vi "Dialog_LogPack (SubVI).vi"() -> ()   [LabVIEW 2017]
uses:
  <vilib>/Utility/miscctls.llb/LVRowAndColumnTypeDef.ctl
  GlobalLog.vi
  <vilib>/Utility/file.llb/Write Delimited Spreadsheet (string).vi
panel:
  in  "Export":bool
  out "Slide":u8(slide) scale=0.0..100.0
  in  "Reload":bool
  in  "Cancel":bool
  in  "OK":bool
  out "Table":string[][](table) caption="Принятые пакеты, Такт 1 ПЭП1...8"
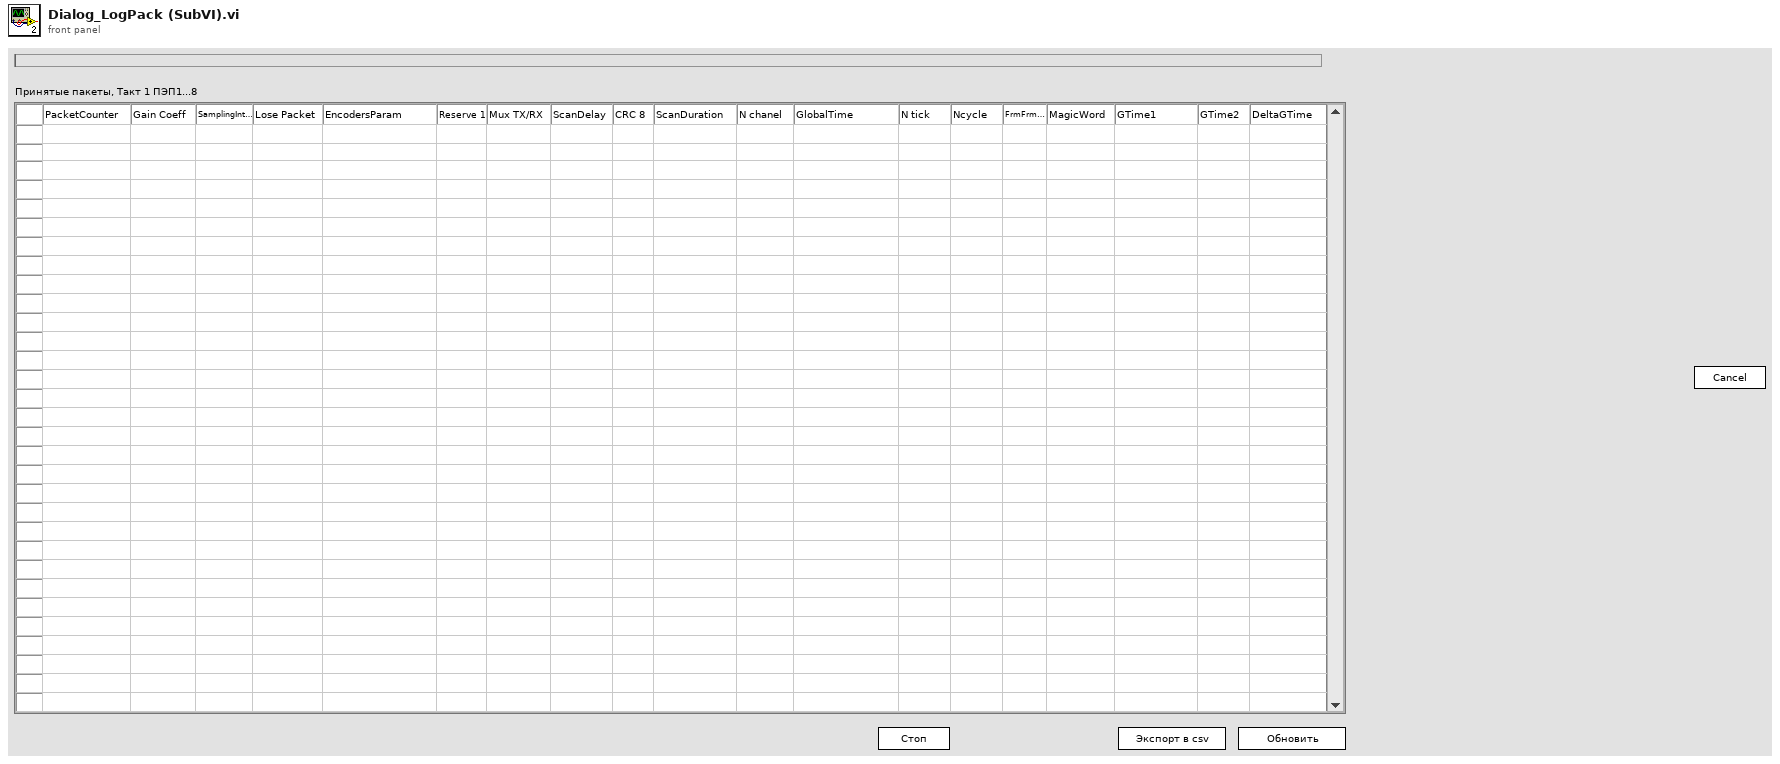
[diagram p1: front panel]
types:
  T1 = typedef "LVRowAndColumnTypeDef.ctl" = cluster{"Row":i32, "Column":i32}
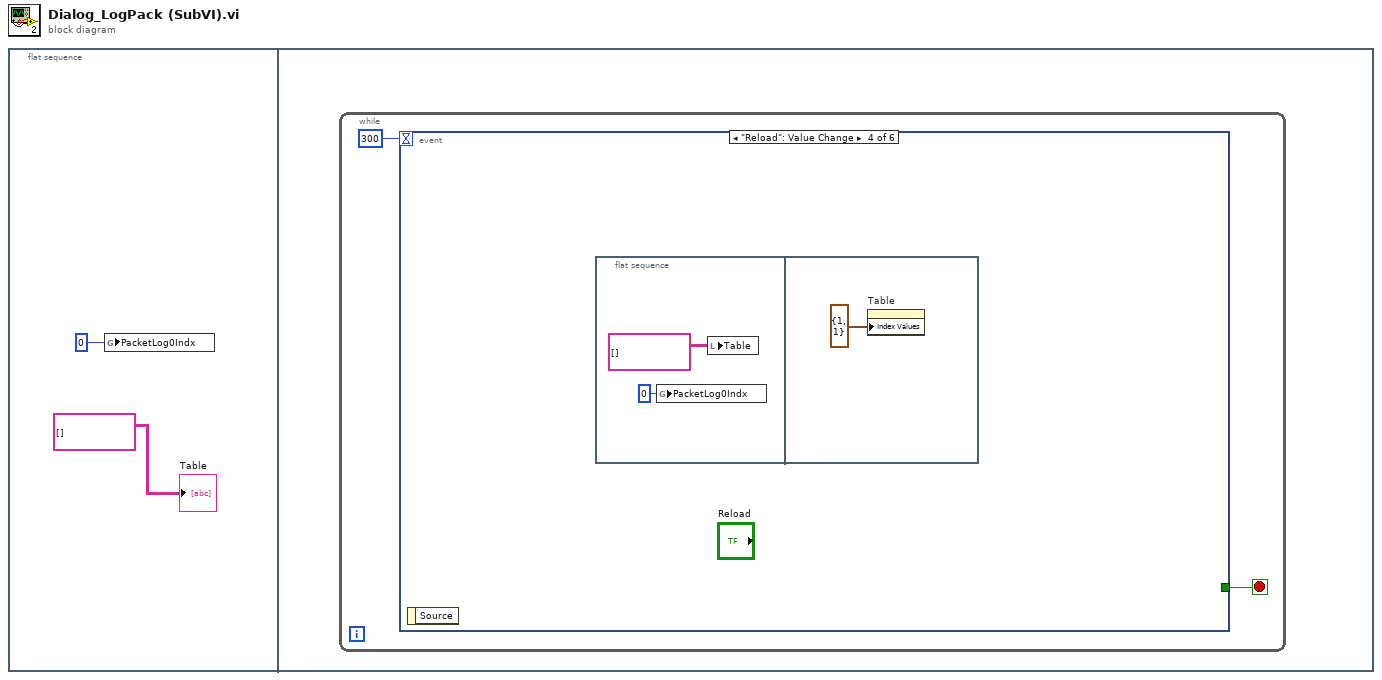
[diagram p0: block diagram]
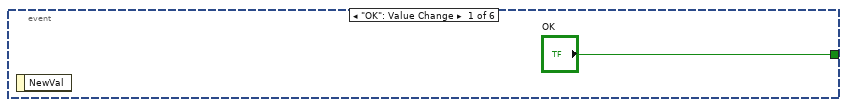
[diagram p2: hidden frame]
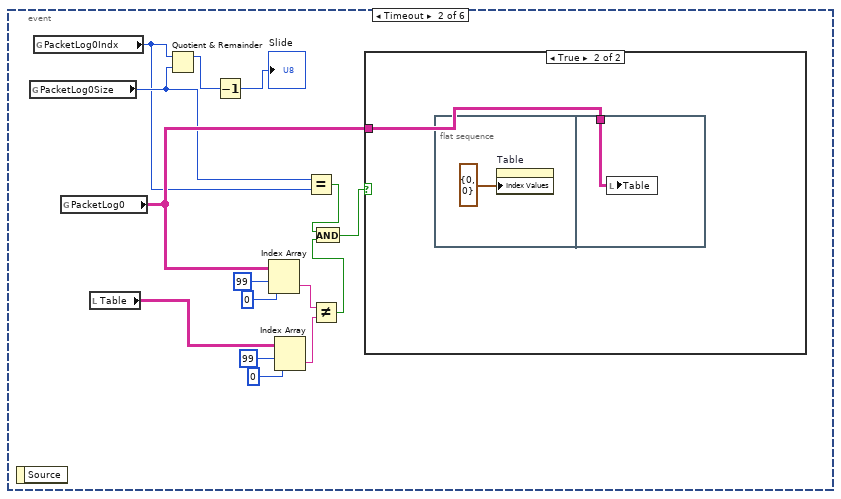
[diagram p3: hidden frame]
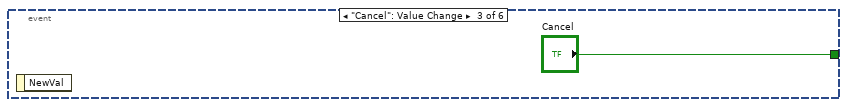
[diagram p5: hidden frame]
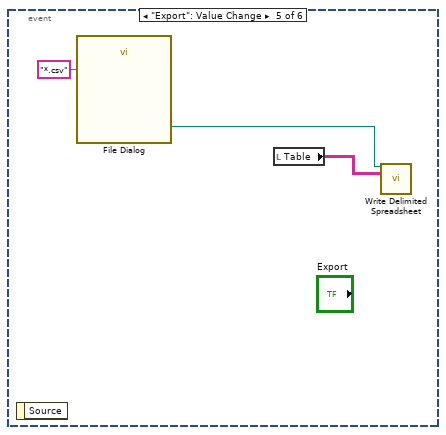
[diagram p6: hidden frame]
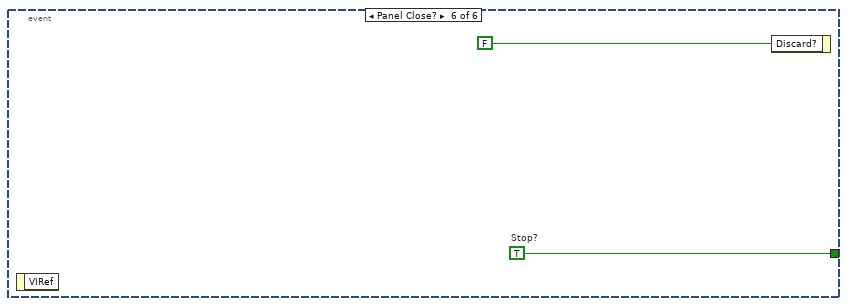
[diagram p7: hidden frame]
diagram:
  n1 = flat-sequence {
    frame #0 {
      n2 = global write "GlobalLog.vi" "PacketLog0Indx"(0 ("PacketLog0Indx")) -> ()
      "Table" <- string[][] [] ("Table")
    }
    frame #1 {
      n3 = while {
        stop <- w3 stop-if-true
        n4 = event shown="[3] \"Reload\": Value Change" {
          selector: _ -> [_ _ _ _ _ _]
          dyn-events: _ -> [_ _ _ _ _ _]
          timeout: 300 -> [_ _ _ _ _ _]
          tunnel: ["OK" _ "Cancel" _ _ w31] -> w3
          event "OK": Value Change {
            n5 = event-data() -> ()  [unwired: 1 in, 1 out]
          }
          event Timeout {
            n6 = event-data() -> ()  [unwired: 1 in, 1 out]
            n7 = global read "GlobalLog.vi" "PacketLog0Size"() -> (w10:i32)
            n8 = global read "GlobalLog.vi" "PacketLog0Indx"() -> (w6:i32)
            n9 = global read "GlobalLog.vi" "PacketLog0"() -> (w11:string[][])
            n10 = local read "Table"() -> (w18:string[][])
            n11 = Quotient & Remainder(x=w6, y=w10) -> (x-y*floor(x/y)=w13:i32)  [unwired: 1 out]
            n12 = Decrement(x=w13) -> (x-1=→"Slide":i32)
            n13 = Index Array(array=w11, index (row)=99, index (col)=0 ("disabled index (col)")) -> (element=w15:string)
            n14 = Index Array(array=w18, index (row)=99, index (col)=0 ("disabled index (col)")) -> (element=w14:string)
            n15 = Equal?(x=w10, y=w6) -> (x = y?=w9:bool)
            n16 = Not Equal?(x=w15, y=w14) -> (x != y?=w8:bool)
            n17 = And(x=w9, y=w8) -> (x .and. y?=w7:bool)
            n18 = case shown="True" w7 {
              tunnel: w11 -> [_ w21]
              frame False {
              }
              frame True {
                n19 = flat-sequence {
                  tunnel: w21 -> [w23]
                  frame #0 {
                    n20 = property on="Table" class="Tbl (strict)"("Index Values"=T1 {"Row"=0, "Column"=0} ("Active Cell:Active Cell")) -> ()  [unwired: 2 in, 2 out]
                  }
                  frame #1 {
                    n21 = local write "Table"(w23) -> ()
                  }
                }
              }
            }
          }
          event "Cancel": Value Change {
            n22 = event-data() -> ()  [unwired: 1 in, 1 out]
          }
          event "Reload": Value Change {
            n23 = event-data() -> ()  [unwired: 1 in, 1 out]
            n24 = flat-sequence {
              frame #0 {
                n25 = global write "GlobalLog.vi" "PacketLog0Indx"(0 ("PacketLog0Indx")) -> ()
                n26 = local write "Table"(string[][] [] ("Table")) -> ()
              }
              frame #1 {
                n27 = property on="Table" class="Tbl (strict)"("Index Values"=T1 {"Row"=1, "Column"=1} ("Active Cell:Active Cell")) -> ()  [unwired: 2 in, 2 out]
              }
            }
          }
          event "Export": Value Change {
            n28 = event-data() -> ()  [unwired: 1 in, 1 out]
            n29 = call "File Dialog"("pattern (all files)"="*.csv") -> ("selected path"=w28:path)  [unwired: 11 in, 3 out]
            n30 = local read "Table"() -> (w30:string[][])
            n31 = call-poly <vilib>:"Write Delimited Spreadsheet.vi"("file path (dialog if empty)"=w28, "2D data"=w30) -> ()  [unwired: 12 in, 2 out]
          }
          event Panel Close? {
            w31 = TRUE  # Stop?
            n32 = event-data() -> ()  [unwired: 1 in, 1 out]
            n33 = event-data("Discard?"=FALSE) -> ()  [unwired: 1 in, 1 out]
          }
        }
      }
    }
  }
